vi "SSL Detection Robots Invalidate.vi"(11 "Robots":T1[](array[typedef]) {"height" format="%+4.3f"; "pixel_y" format="%+4.3f"; "pixel_x" format="%+4.3f"; "orientation" format="%+4.3f"; "y" format="%+4.3f"; "confidence" format="%4.3f"; "x" format="%+4.3f"}) -> (2 "Indexes":u32[](array[numeric]), 3 "Robots Invalidated":T1[](array[typedef]) {"height" format="%+4.3f"; "pixel_y" format="%+4.3f"; "pixel_x" format="%+4.3f"; "orientation" format="%+4.3f"; "y" format="%+4.3f"; "confidence" format="%4.3f"; "x" format="%+4.3f"})   [LabVIEW 2016]
uses:
  SSL Detection Robot.ctl
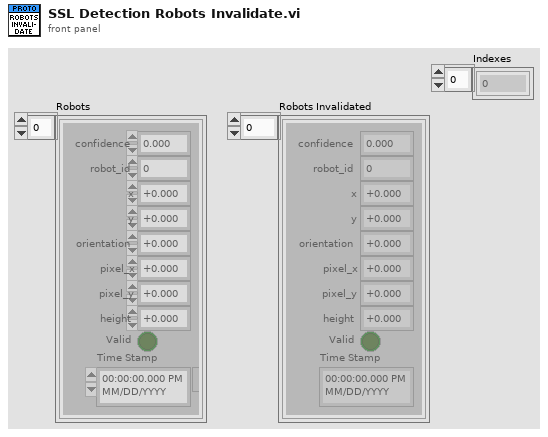
[diagram p1: front panel]
types:
  T1 = typedef "SSL Detection Robot.ctl" = cluster{"x":dbl, "robot_id":u32, "confidence":sgl, "y":sgl, "orientation":sgl, "pixel_x":sgl, "pixel_y":sgl, "height":sgl, "Valid":bool, "Time Stamp":timestamp}
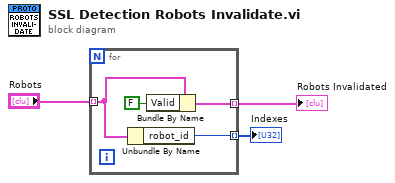
[diagram p0: block diagram]
diagram:
  n1 = for {
    tunnel: "Robots" -> [w5] mode=indexing
    tunnel: [w6] -> w3 mode=indexing
    tunnel: [w4] -> w1 mode=indexing
    n2 = Unbundle By Name(w5) -> ("robot_id"=w4:u32)
    n3 = Bundle By Name(cluster=w5, "Valid"=FALSE) -> (w6:T1)
  }
  "Robots Invalidated" <- w3
  "Indexes" <- w1
